vi "generateBlobs.vi"(6 "timeout (10000)":i32=10000, 8 "error in (no error)":errorcluster, 11 "Parameters":T2={"params"={"apiKey"="", "n"=0, "size"=0, "format"="base64"}, "id"=0.0}) -> (0 "error out":errorcluster, 3 "Response":T1, 4 "error data":string[](array[string]))   [LabVIEW 2014, in "Random JSON API.lvlib"]
uses:
  Random JSON API.lvlib
  Type Defs/generateBlobsRequest.ctl
  Type Defs/generateBlobsResponse.ctl
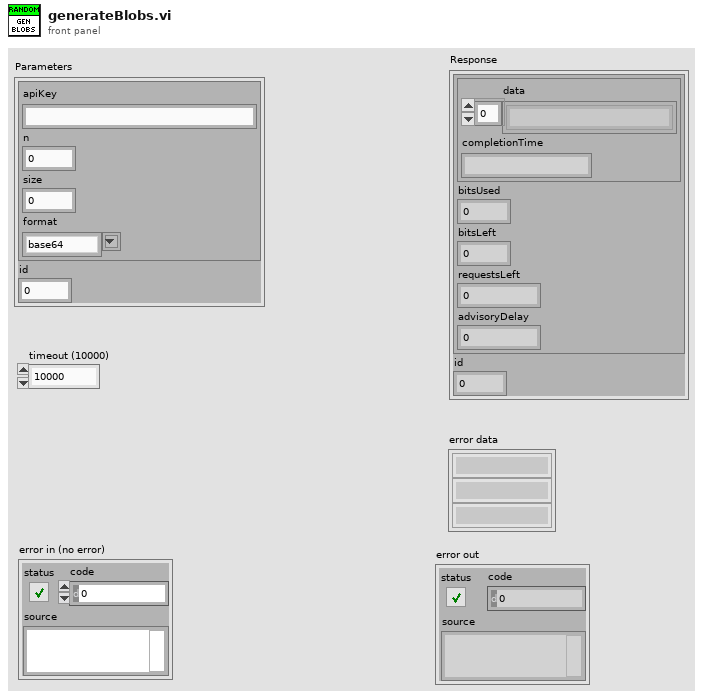
[diagram p1: front panel]
types:
  T1 = typedef "Random JSON API.lvlib/generateBlobsResponse.ctl" = cluster{"result":cluster{"random":cluster{"data":string[], "completionTime":string}, "bitsUsed":i32, "bitsLeft":i32, "requestsLeft":i32, "advisoryDelay":i32}, "id":dbl}
  T2 = typedef "Random JSON API.lvlib/generateBlobsRequest.ctl" = cluster{"params":cluster{"apiKey":string, "n":i32, "size":i32, "format":string}, "id":dbl}
  T3 = cluster{"apiKey":string, "n":i32, "size":i32, "format":string}
  T4 = cluster{"jsonrpc":string, "method":string, "params":cluster{"apiKey":string, "n":i32, "size":i32, "format":string}, "id":dbl}
  T5 = cluster{"completionTime":string, "bitsUsed":i32, "bitsLeft":i32, "requestsLeft":i32, "advisoryDelay":i32}
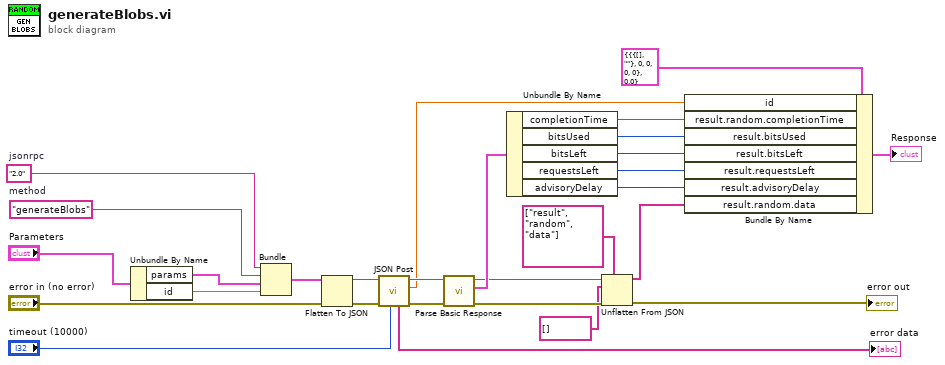
[diagram p0: block diagram]
diagram:
  w14 = "2.0"  # jsonrpc
  w19 = "generateBlobs"  # method
  n1 = Unbundle By Name("Parameters") -> ("params"=w17:T3, "id"=w16:dbl)
  n2 = Bundle("jsonrpc"=w14, "method"=w19, "params"=w17, "id"=w16) -> (w15:T4)  [unwired: 1 in]
  n3 = Flatten To JSON(anything=w15, error in (no error)="error in (no error)") -> (JSON string=w20:string, 11:w21:errorcluster)  [unwired: 1 in]
  n4 = call "JSON Post.vi"("timeout (10000)"="timeout (10000)", "error in (no error)"=w21, "Request JSON String"=w20) -> ("error out"=w28:errorcluster, "id"=w12:dbl, "Response JSON String"=w13:string, "error data"=→"error data":string[])  [unwired: 5 in]
  n5 = call "Parse Basic Response.vi"("error in (no error)"=w28, "body in"=w13) -> ("error out"=w10:errorcluster, "result cluster"=w11:T5, "body out"=w8:string)  [unwired: 7 in]
  n6 = Unbundle By Name(w11) -> ("completionTime"=w27:string, "bitsUsed"=w26:i32, "bitsLeft"=w25:i32, "requestsLeft"=w24:i32, "advisoryDelay"=w23:i32)
  n7 = Unflatten From JSON(path=string[] ["result", "random", "data"], JSON string=w8, type and defaults=string[] [], error in (no error)=w10) -> (value=w6:string[], error out=→"error out":errorcluster)  [unwired: 3 in]
  n8 = Bundle By Name(cluster=T1 {"result"={"random"={"data"=[], "completionTime"=""}, "bitsUsed"=0, "bitsLeft"=0, "requestsLeft"=0, "advisoryDelay"=0}, "id"=0.0} ("Response"), "id"=w12, "result.random.completionTime"=w27, "result.bitsUsed"=w26, "result.bitsLeft"=w25, "result.requestsLeft"=w24, "result.advisoryDelay"=w23, "result.random.data"=w6) -> (→"Response":T1)
